vi "MaxZ_FITSstacks.vi"() -> ()   [LabVIEW 2011]
panel:
  out "error out":errorcluster
  in  "intensity scale factor":dbl=8.0
  out "plane#":i32=24
  out "Intensity Graph":u16[][](graph)
  in  "output folder for 16bit TIFs":path=path "D:/freigabe/Max"
  out "fits#":i32=365
  in  "All Files in Dir":path[](array[path])=[path "E:/Auswertung_ISS/002_2018-06-21_16-44-14/raw_I000_X0_C0.fits.EPI.fits", path "E:/Auswertung_ISS/002_2018-06-21_16-44-14/raw_I000_X0_C1.fits.EPI.fits", path "E:/Auswertung_ISS/002_2018-06-21_16-44-14/raw_I000_X0_C3.fits.EPI.fits", path "E:/Auswertung_ISS/002_2018-06-21_16-44-14/raw_I000_X1_C0.fits.EPI.fits", path "E:/Auswertung_ISS/002_2018-06-21_16-44-14/raw_I000_X1_C3.fits.EPI.fits", path "E:/Auswertung_ISS/003_2018-07-03_15-08-29/raw_I000_X0_C0.fits.EPI.fits", path "E:/Auswertung_ISS/003_2018-07-03_15-08-29/raw_I000_X0_C1.fits.EPI.fits", path "E:/Auswertung_ISS/003_2018-07-03_15-08-29/raw_I000_X0_C3.fits.EPI.fits", path "E:/Auswertung_ISS/003_2018-07-03_15-08-29/raw_I000_X1_C0.fits.EPI.fits", path "E:/Auswertung_ISS/003_2018-07-03_15-08-29/raw_I000_X1_C3.fits.EPI.fits", path "E:/Auswertung_ISS/003_2018-07-03_15-08-29/raw_I001_X1_C0.fits.EPI.fits", path "E:/Auswertung_ISS/003_2018-07-03_15-08-29/raw_I001_X1_C3.fits.EPI.fits", path "E:/Auswertung_ISS/003_2018-07-03_15-08-29/raw_I002_X1_C0.fits.EPI.fits", path "E:/Auswertung_ISS/003_2018-07-03_15-08-29/raw_I002_X1_C3.fits.EPI.fits", path "E:/Auswertung_ISS/003_2018-07-03_15-08-29/raw_I003_X1_C0.fits.EPI.fits", path "E:/Auswertung_ISS/003_2018-07-03_15-08-29/raw_I003_X1_C3.fits.EPI.fits", path "E:/Auswertung_ISS/003_2018-07-03_15-08-29/raw_I004_X1_C0.fits.EPI.fits", path "E:/Auswertung_ISS/003_2018-07-03_15-08-29/raw_I004_X1_C3.fits.EPI.fits", path "E:/Auswertung_ISS/003_2018-07-03_15-08-29/raw_I005_X1_C0.fits.EPI.fits", path "E:/Auswertung_ISS/003_2018-07-03_15-08-29/raw_I005_X1_C3.fits.EPI.fits", path "E:/Auswertung_ISS/003_2018-07-03_15-08-29/raw_I006_X1_C0.fits.EPI.fits", path "E:/Auswertung_ISS/003_2018-07-03_15-08-29/raw_I006_X1_C3.fits.EPI.fits", path "E:/Auswertung_ISS/003_2018-07-03_15-08-29/raw_I007_X1_C0.fits.EPI.fits", path "E:/Auswertung_ISS/003_2018-07-03_15-08-29/raw_I007_X1_C3.fits.EPI.fits", path "E:/Auswertung_ISS/003_2018-07-03_15-08-29/raw_I008_X1_C0.fits.EPI.fits", path "E:/Auswertung_ISS/003_2018-07-03_15-08-29/raw_I008_X1_C3.fits.EPI.fits", path "E:/Auswertung_ISS/003_2018-07-03_15-08-29/raw_I009_X0_C0.fits.EPI.fits", path "E:/Auswertung_ISS/003_2018-07-03_15-08-29/raw_I009_X0_C1.fits.EPI.fits", path "E:/Auswertung_ISS/003_2018-07-03_15-08-29/raw_I009_X0_C3.fits.EPI.fits", path "E:/Auswertung_ISS/003_2018-07-03_15-08-29/raw_I009_X1_C0.fits.EPI.fits", path "E:/Auswertung_ISS/003_2018-07-03_15-08-29/raw_I009_X1_C3.fits.EPI.fits", path "E:/Auswertung_ISS/004_2018-07-03_17-33-15/raw_I000_X0_C0.fits.EPI.fits", path "E:/Auswertung_ISS/004_2018-07-03_17-33-15/raw_I000_X0_C1.fits.EPI.fits", path "E:/Auswertung_ISS/004_2018-07-03_17-33-15/raw_I000_X0_C3.fits.EPI.fits", path "E:/Auswertung_ISS/004_2018-07-03_17-33-15/raw_I000_X1_C0.fits.EPI.fits", path "E:/Auswertung_ISS/004_2018-07-03_17-33-15/raw_I000_X1_C3.fits.EPI.fits", path "E:/Auswertung_ISS/004_2018-07-03_17-33-15/raw_I001_X1_C0.fits.EPI.fits", path "E:/Auswertung_ISS/004_2018-07-03_17-33-15/raw_I001_X1_C3.fits.EPI.fits", path "E:/Auswertung_ISS/004_2018-07-03_17-33-15/raw_I002_X1_C0.fits.EPI.fits", path "E:/Auswertung_ISS/004_2018-07-03_17-33-15/raw_I002_X1_C3.fits.EPI.fits", path "E:/Auswertung_ISS/004_2018-07-03_17-33-15/raw_I003_X1_C0.fits.EPI.fits", path "E:/Auswertung_ISS/004_2018-07-03_17-33-15/raw_I003_X1_C3.fits.EPI.fits", path "E:/Auswertung_ISS/004_2018-07-03_17-33-15/raw_I004_X1_C0.fits.EPI.fits", path "E:/Auswertung_ISS/004_2018-07-03_17-33-15/raw_I004_X1_C3.fits.EPI.fits", path "E:/Auswertung_ISS/004_2018-07-03_17-33-15/raw_I005_X1_C0.fits.EPI.fits", path "E:/Auswertung_ISS/004_2018-07-03_17-33-15/raw_I005_X1_C3.fits.EPI.fits", path "E:/Auswertung_ISS/004_2018-07-03_17-33-15/raw_I006_X1_C0.fits.EPI.fits", path "E:/Auswertung_ISS/004_2018-07-03_17-33-15/raw_I006_X1_C3.fits.EPI.fits", path "E:/Auswertung_ISS/004_2018-07-03_17-33-15/raw_I007_X1_C0.fits.EPI.fits", path "E:/Auswertung_ISS/004_2018-07-03_17-33-15/raw_I007_X1_C3.fits.EPI.fits", path "E:/Auswertung_ISS/004_2018-07-03_17-33-15/raw_I008_X1_C0.fits.EPI.fits", path "E:/Auswertung_ISS/004_2018-07-03_17-33-15/raw_I008_X1_C3.fits.EPI.fits", path "E:/Auswertung_ISS/004_2018-07-03_17-33-15/raw_I009_X1_C0.fits.EPI.fits", path "E:/Auswertung_ISS/004_2018-07-03_17-33-15/raw_I009_X1_C3.fits.EPI.fits", path "E:/Auswertung_ISS/004_2018-07-03_17-33-15/raw_I010_X1_C0.fits.EPI.fits", path "E:/Auswertung_ISS/004_2018-07-03_17-33-15/raw_I010_X1_C3.fits.EPI.fits", path "E:/Auswertung_ISS/004_2018-07-03_17-33-15/raw_I011_X1_C0.fits.EPI.fits", path "E:/Auswertung_ISS/004_2018-07-03_17-33-15/raw_I011_X1_C3.fits.EPI.fits", path "E:/Auswertung_ISS/004_2018-07-03_17-33-15/raw_I012_X1_C0.fits.EPI.fits", path "E:/Auswertung_ISS/004_2018-07-03_17-33-15/raw_I012_X1_C3.fits.EPI.fits", path "E:/Auswertung_ISS/004_2018-07-03_17-33-15/raw_I013_X1_C0.fits.EPI.fits", path "E:/Auswertung_ISS/004_2018-07-03_17-33-15/raw_I013_X1_C3.fits.EPI.fits", path "E:/Auswertung_ISS/004_2018-07-03_17-33-15/raw_I014_X1_C0.fits.EPI.fits", path "E:/Auswertung_ISS/004_2018-07-03_17-33-15/raw_I014_X1_C3.fits.EPI.fits", path "E:/Auswertung_ISS/004_2018-07-03_17-33-15/raw_I015_X1_C0.fits.EPI.fits", path "E:/Auswertung_ISS/004_2018-07-03_17-33-15/raw_I015_X1_C3.fits.EPI.fits", path "E:/Auswertung_ISS/004_2018-07-03_17-33-15/raw_I016_X1_C0.fits.EPI.fits", path "E:/Auswertung_ISS/004_2018-07-03_17-33-15/raw_I016_X1_C3.fits.EPI.fits", path "E:/Auswertung_ISS/004_2018-07-03_17-33-15/raw_I017_X1_C0.fits.EPI.fits", path "E:/Auswertung_ISS/004_2018-07-03_17-33-15/raw_I017_X1_C3.fits.EPI.fits", path "E:/Auswertung_ISS/005_2018-07-04_08-02-54/raw_I000_X0_C0.fits.EPI.fits", path "E:/Auswertung_ISS/005_2018-07-04_08-02-54/raw_I000_X0_C1.fits.EPI.fits", path "E:/Auswertung_ISS/005_2018-07-04_08-02-54/raw_I000_X0_C3.fits.EPI.fits", path "E:/Auswertung_ISS/005_2018-07-04_08-02-54/raw_I000_X1_C0.fits.EPI.fits", path "E:/Auswertung_ISS/005_2018-07-04_08-02-54/raw_I000_X1_C3.fits.EPI.fits", path "E:/Auswertung_ISS/005_2018-07-04_08-02-54/raw_I001_X1_C0.fits.EPI.fits", path "E:/Auswertung_ISS/005_2018-07-04_08-02-54/raw_I001_X1_C3.fits.EPI.fits", path "E:/Auswertung_ISS/005_2018-07-04_08-02-54/raw_I002_X1_C0.fits.EPI.fits", path "E:/Auswertung_ISS/005_2018-07-04_08-02-54/raw_I002_X1_C3.fits.EPI.fits", path "E:/Auswertung_ISS/005_2018-07-04_08-02-54/raw_I003_X1_C0.fits.EPI.fits", path "E:/Auswertung_ISS/005_2018-07-04_08-02-54/raw_I003_X1_C3.fits.EPI.fits", path "E:/Auswertung_ISS/005_2018-07-04_08-02-54/raw_I004_X1_C0.fits.EPI.fits", path "E:/Auswertung_ISS/005_2018-07-04_08-02-54/raw_I004_X1_C3.fits.EPI.fits", path "E:/Auswertung_ISS/005_2018-07-04_08-02-54/raw_I005_X1_C0.fits.EPI.fits", path "E:/Auswertung_ISS/005_2018-07-04_08-02-54/raw_I005_X1_C3.fits.EPI.fits", path "E:/Auswertung_ISS/005_2018-07-04_08-02-54/raw_I006_X1_C0.fits.EPI.fits", path "E:/Auswertung_ISS/005_2018-07-04_08-02-54/raw_I006_X1_C3.fits.EPI.fits", path "E:/Auswertung_ISS/005_2018-07-04_08-02-54/raw_I007_X1_C0.fits.EPI.fits", path "E:/Auswertung_ISS/005_2018-07-04_08-02-54/raw_I007_X1_C3.fits.EPI.fits", path "E:/Auswertung_ISS/005_2018-07-04_08-02-54/raw_I008_X1_C0.fits.EPI.fits", path "E:/Auswertung_ISS/005_2018-07-04_08-02-54/raw_I008_X1_C3.fits.EPI.fits", path "E:/Auswertung_ISS/005_2018-07-04_08-02-54/raw_I009_X1_C0.fits.EPI.fits", path "E:/Auswertung_ISS/005_2018-07-04_08-02-54/raw_I009_X1_C3.fits.EPI.fits", path "E:/Auswertung_ISS/005_2018-07-04_08-02-54/raw_I010_X1_C0.fits.EPI.fits", path "E:/Auswertung_ISS/005_2018-07-04_08-02-54/raw_I010_X1_C3.fits.EPI.fits", path "E:/Auswertung_ISS/005_2018-07-04_08-02-54/raw_I011_X1_C0.fits.EPI.fits", path "E:/Auswertung_ISS/005_2018-07-04_08-02-54/raw_I011_X1_C3.fits.EPI.fits", path "E:/Auswertung_ISS/005_2018-07-04_08-02-54/raw_I012_X1_C0.fits.EPI.fits", path "E:/Auswertung_ISS/005_2018-07-04_08-02-54/raw_I012_X1_C3.fits.EPI.fits", path "E:/Auswertung_ISS/005_2018-07-04_08-02-54/raw_I013_X1_C0.fits.EPI.fits", path "E:/Auswertung_ISS/005_2018-07-04_08-02-54/raw_I013_X1_C3.fits.EPI.fits", path "E:/Auswertung_ISS/005_2018-07-04_08-02-54/raw_I014_X1_C0.fits.EPI.fits", path "E:/Auswertung_ISS/005_2018-07-04_08-02-54/raw_I014_X1_C3.fits.EPI.fits", path "E:/Auswertung_ISS/005_2018-07-04_08-02-54/raw_I015_X1_C0.fits.EPI.fits", path "E:/Auswertung_ISS/005_2018-07-04_08-02-54/raw_I015_X1_C3.fits.EPI.fits", path "E:/Auswertung_ISS/005_2018-07-04_08-02-54/raw_I016_X1_C0.fits.EPI.fits", path "E:/Auswertung_ISS/005_2018-07-04_08-02-54/raw_I016_X1_C3.fits.EPI.fits", path "E:/Auswertung_ISS/006_2018-07-04_15-43-18/raw_I000_X0_C0.fits.EPI.fits", path "E:/Auswertung_ISS/006_2018-07-04_15-43-18/raw_I000_X0_C1.fits.EPI.fits", path "E:/Auswertung_ISS/006_2018-07-04_15-43-18/raw_I000_X0_C3.fits.EPI.fits", path "E:/Auswertung_ISS/006_2018-07-04_15-43-18/raw_I000_X1_C0.fits.EPI.fits", path "E:/Auswertung_ISS/006_2018-07-04_15-43-18/raw_I000_X1_C3.fits.EPI.fits", path "E:/Auswertung_ISS/006_2018-07-04_15-43-18/raw_I001_X1_C0.fits.EPI.fits", path "E:/Auswertung_ISS/006_2018-07-04_15-43-18/raw_I001_X1_C3.fits.EPI.fits", path "E:/Auswertung_ISS/006_2018-07-04_15-43-18/raw_I002_X1_C0.fits.EPI.fits", path "E:/Auswertung_ISS/006_2018-07-04_15-43-18/raw_I002_X1_C3.fits.EPI.fits", path "E:/Auswertung_ISS/006_2018-07-04_15-43-18/raw_I003_X1_C0.fits.EPI.fits", path "E:/Auswertung_ISS/006_2018-07-04_15-43-18/raw_I003_X1_C3.fits.EPI.fits", path "E:/Auswertung_ISS/007_2018-07-04_16-44-22/raw_I000_X0_C0.fits.EPI.fits", path "E:/Auswertung_ISS/007_2018-07-04_16-44-22/raw_I000_X0_C1.fits.EPI.fits", path "E:/Auswertung_ISS/007_2018-07-04_16-44-22/raw_I000_X0_C3.fits.EPI.fits", path "E:/Auswertung_ISS/007_2018-07-04_16-44-22/raw_I000_X1_C0.fits.EPI.fits", path "E:/Auswertung_ISS/007_2018-07-04_16-44-22/raw_I000_X1_C3.fits.EPI.fits", path "E:/Auswertung_ISS/007_2018-07-04_16-44-22/raw_I001_X1_C0.fits.EPI.fits", path "E:/Auswertung_ISS/007_2018-07-04_16-44-22/raw_I001_X1_C3.fits.EPI.fits", path "E:/Auswertung_ISS/007_2018-07-04_16-44-22/raw_I002_X1_C0.fits.EPI.fits", path "E:/Auswertung_ISS/007_2018-07-04_16-44-22/raw_I002_X1_C3.fits.EPI.fits", path "E:/Auswertung_ISS/007_2018-07-04_16-44-22/raw_I003_X1_C0.fits.EPI.fits", path "E:/Auswertung_ISS/007_2018-07-04_16-44-22/raw_I003_X1_C3.fits.EPI.fits", path "E:/Auswertung_ISS/007_2018-07-04_16-44-22/raw_I004_X1_C0.fits.EPI.fits", path "E:/Auswertung_ISS/007_2018-07-04_16-44-22/raw_I004_X1_C3.fits.EPI.fits", path "E:/Auswertung_ISS/007_2018-07-04_16-44-22/raw_I005_X1_C0.fits.EPI.fits", path "E:/Auswertung_ISS/007_2018-07-04_16-44-22/raw_I005_X1_C3.fits.EPI.fits", path "E:/Auswertung_ISS/007_2018-07-04_16-44-22/raw_I006_X1_C0.fits.EPI.fits", path "E:/Auswertung_ISS/007_2018-07-04_16-44-22/raw_I006_X1_C3.fits.EPI.fits", path "E:/Auswertung_ISS/007_2018-07-04_16-44-22/raw_I007_X1_C0.fits.EPI.fits", path "E:/Auswertung_ISS/007_2018-07-04_16-44-22/raw_I007_X1_C3.fits.EPI.fits", path "E:/Auswertung_ISS/007_2018-07-04_16-44-22/raw_I008_X1_C0.fits.EPI.fits", path "E:/Auswertung_ISS/007_2018-07-04_16-44-22/raw_I008_X1_C3.fits.EPI.fits", path "E:/Auswertung_ISS/007_2018-07-04_16-44-22/raw_I009_X1_C0.fits.EPI.fits", path "E:/Auswertung_ISS/007_2018-07-04_16-44-22/raw_I009_X1_C3.fits.EPI.fits", path "E:/Auswertung_ISS/007_2018-07-04_16-44-22/raw_I010_X1_C0.fits.EPI.fits", path "E:/Auswertung_ISS/007_2018-07-04_16-44-22/raw_I010_X1_C3.fits.EPI.fits", path "E:/Auswertung_ISS/007_2018-07-04_16-44-22/raw_I011_X1_C0.fits.EPI.fits", path "E:/Auswertung_ISS/007_2018-07-04_16-44-22/raw_I011_X1_C3.fits.EPI.fits", path "E:/Auswertung_ISS/007_2018-07-04_16-44-22/raw_I012_X1_C0.fits.EPI.fits", path "E:/Auswertung_ISS/007_2018-07-04_16-44-22/raw_I012_X1_C3.fits.EPI.fits", path "E:/Auswertung_ISS/007_2018-07-04_16-44-22/raw_I013_X1_C0.fits.EPI.fits", path "E:/Auswertung_ISS/007_2018-07-04_16-44-22/raw_I013_X1_C3.fits.EPI.fits", path "E:/Auswertung_ISS/007_2018-07-04_16-44-22/raw_I014_X1_C0.fits.EPI.fits", path "E:/Auswertung_ISS/007_2018-07-04_16-44-22/raw_I014_X1_C3.fits.EPI.fits", path "E:/Auswertung_ISS/007_2018-07-04_16-44-22/raw_I015_X1_C0.fits.EPI.fits", path "E:/Auswertung_ISS/007_2018-07-04_16-44-22/raw_I015_X1_C3.fits.EPI.fits", path "E:/Auswertung_ISS/007_2018-07-04_16-44-22/raw_I016_X1_C0.fits.EPI.fits", path "E:/Auswertung_ISS/007_2018-07-04_16-44-22/raw_I016_X1_C3.fits.EPI.fits", path "E:/Auswertung_ISS/007_2018-07-04_16-44-22/raw_I017_X1_C0.fits.EPI.fits", path "E:/Auswertung_ISS/007_2018-07-04_16-44-22/raw_I017_X1_C3.fits.EPI.fits", path "E:/Auswertung_ISS/008_2018-07-05_08-02-52/raw_I000_X0_C0.fits.EPI.fits", path "E:/Auswertung_ISS/008_2018-07-05_08-02-52/raw_I000_X0_C1.fits.EPI.fits", path "E:/Auswertung_ISS/008_2018-07-05_08-02-52/raw_I000_X0_C3.fits.EPI.fits", path "E:/Auswertung_ISS/008_2018-07-05_08-02-52/raw_I000_X1_C0.fits.EPI.fits", path "E:/Auswertung_ISS/008_2018-07-05_08-02-52/raw_I000_X1_C3.fits.EPI.fits", path "E:/Auswertung_ISS/008_2018-07-05_08-02-52/raw_I001_X1_C0.fits.EPI.fits", path "E:/Auswertung_ISS/008_2018-07-05_08-02-52/raw_I001_X1_C3.fits.EPI.fits", path "E:/Auswertung_ISS/008_2018-07-05_08-02-52/raw_I002_X1_C0.fits.EPI.fits", path "E:/Auswertung_ISS/008_2018-07-05_08-02-52/raw_I002_X1_C3.fits.EPI.fits", path "E:/Auswertung_ISS/008_2018-07-05_08-02-52/raw_I003_X1_C0.fits.EPI.fits", path "E:/Auswertung_ISS/008_2018-07-05_08-02-52/raw_I003_X1_C3.fits.EPI.fits", path "E:/Auswertung_ISS/008_2018-07-05_08-02-52/raw_I004_X1_C0.fits.EPI.fits", path "E:/Auswertung_ISS/008_2018-07-05_08-02-52/raw_I004_X1_C3.fits.EPI.fits", path "E:/Auswertung_ISS/008_2018-07-05_08-02-52/raw_I005_X1_C0.fits.EPI.fits", path "E:/Auswertung_ISS/008_2018-07-05_08-02-52/raw_I005_X1_C3.fits.EPI.fits", path "E:/Auswertung_ISS/008_2018-07-05_08-02-52/raw_I006_X1_C0.fits.EPI.fits", path "E:/Auswertung_ISS/008_2018-07-05_08-02-52/raw_I006_X1_C3.fits.EPI.fits", path "E:/Auswertung_ISS/008_2018-07-05_08-02-52/raw_I007_X1_C0.fits.EPI.fits", path "E:/Auswertung_ISS/008_2018-07-05_08-02-52/raw_I007_X1_C3.fits.EPI.fits", path "E:/Auswertung_ISS/008_2018-07-05_08-02-52/raw_I008_X1_C0.fits.EPI.fits", path "E:/Auswertung_ISS/008_2018-07-05_08-02-52/raw_I008_X1_C3.fits.EPI.fits", path "E:/Auswertung_ISS/008_2018-07-05_08-02-52/raw_I009_X1_C0.fits.EPI.fits", path "E:/Auswertung_ISS/008_2018-07-05_08-02-52/raw_I009_X1_C3.fits.EPI.fits", path "E:/Auswertung_ISS/008_2018-07-05_08-02-52/raw_I010_X1_C0.fits.EPI.fits", path "E:/Auswertung_ISS/008_2018-07-05_08-02-52/raw_I010_X1_C3.fits.EPI.fits", path "E:/Auswertung_ISS/008_2018-07-05_08-02-52/raw_I011_X1_C0.fits.EPI.fits", path "E:/Auswertung_ISS/008_2018-07-05_08-02-52/raw_I011_X1_C3.fits.EPI.fits", path "E:/Auswertung_ISS/008_2018-07-05_08-02-52/raw_I012_X1_C0.fits.EPI.fits", path "E:/Auswertung_ISS/008_2018-07-05_08-02-52/raw_I012_X1_C3.fits.EPI.fits", path "E:/Auswertung_ISS/008_2018-07-05_08-02-52/raw_I013_X1_C0.fits.EPI.fits", path "E:/Auswertung_ISS/008_2018-07-05_08-02-52/raw_I013_X1_C3.fits.EPI.fits", path "E:/Auswertung_ISS/008_2018-07-05_08-02-52/raw_I014_X1_C0.fits.EPI.fits", path "E:/Auswertung_ISS/008_2018-07-05_08-02-52/raw_I014_X1_C3.fits.EPI.fits", path "E:/Auswertung_ISS/008_2018-07-05_08-02-52/raw_I015_X1_C0.fits.EPI.fits", path "E:/Auswertung_ISS/008_2018-07-05_08-02-52/raw_I015_X1_C3.fits.EPI.fits", path "E:/Auswertung_ISS/008_2018-07-05_08-02-52/raw_I016_X1_C0.fits.EPI.fits", path "E:/Auswertung_ISS/008_2018-07-05_08-02-52/raw_I016_X1_C3.fits.EPI.fits", path "E:/Auswertung_ISS/008_2018-07-05_08-02-52/raw_I017_X1_C0.fits.EPI.fits", path "E:/Auswertung_ISS/008_2018-07-05_08-02-52/raw_I017_X1_C3.fits.EPI.fits", path "E:/Auswertung_ISS/009_2018-07-05_20-57-36/raw_I000_X0_C0.fits.EPI.fits", path "E:/Auswertung_ISS/009_2018-07-05_20-57-36/raw_I000_X0_C1.fits.EPI.fits", path "E:/Auswertung_ISS/009_2018-07-05_20-57-36/raw_I000_X0_C3.fits.EPI.fits", path "E:/Auswertung_ISS/009_2018-07-05_20-57-36/raw_I000_X1_C3.fits.EPI.fits", path "E:/Auswertung_ISS/009_2018-07-05_20-57-36/raw_I001_X1_C3.fits.EPI.fits", path "E:/Auswertung_ISS/009_2018-07-05_20-57-36/raw_I002_X1_C3.fits.EPI.fits", path "E:/Auswertung_ISS/009_2018-07-05_20-57-36/raw_I003_X1_C3.fits.EPI.fits", path "E:/Auswertung_ISS/009_2018-07-05_20-57-36/raw_I004_X1_C3.fits.EPI.fits", path "E:/Auswertung_ISS/009_2018-07-05_20-57-36/raw_I005_X1_C3.fits.EPI.fits", path "E:/Auswertung_ISS/009_2018-07-05_20-57-36/raw_I006_X1_C3.fits.EPI.fits", path "E:/Auswertung_ISS/009_2018-07-05_20-57-36/raw_I007_X1_C3.fits.EPI.fits", path "E:/Auswertung_ISS/009_2018-07-05_20-57-36/raw_I008_X1_C3.fits.EPI.fits", path "E:/Auswertung_ISS/009_2018-07-05_20-57-36/raw_I009_X1_C3.fits.EPI.fits", path "E:/Auswertung_ISS/009_2018-07-05_20-57-36/raw_I010_X1_C3.fits.EPI.fits", path "E:/Auswertung_ISS/009_2018-07-05_20-57-36/raw_I011_X1_C3.fits.EPI.fits", path "E:/Auswertung_ISS/010_2018-07-06_17-20-26/raw_I000_X0_C0.fits.EPI.fits", path "E:/Auswertung_ISS/010_2018-07-06_17-20-26/raw_I000_X0_C1.fits.EPI.fits", path "E:/Auswertung_ISS/010_2018-07-06_17-20-26/raw_I000_X0_C3.fits.EPI.fits", path "E:/Auswertung_ISS/010_2018-07-06_17-20-26/raw_I000_X1_C3.fits.EPI.fits", path "E:/Auswertung_ISS/010_2018-07-06_17-20-26/raw_I001_X0_C0.fits.EPI.fits", path "E:/Auswertung_ISS/010_2018-07-06_17-20-26/raw_I001_X0_C1.fits.EPI.fits", path "E:/Auswertung_ISS/010_2018-07-06_17-20-26/raw_I001_X0_C3.fits.EPI.fits", path "E:/Auswertung_ISS/011_2018-07-06_17-40-54/raw_I000_X0_C0.fits.EPI.fits", path "E:/Auswertung_ISS/011_2018-07-06_17-40-54/raw_I000_X0_C1.fits.EPI.fits", path "E:/Auswertung_ISS/011_2018-07-06_17-40-54/raw_I000_X0_C3.fits.EPI.fits", path "E:/Auswertung_ISS/011_2018-07-06_17-40-54/raw_I000_X1_C3.fits.EPI.fits", path "E:/Auswertung_ISS/011_2018-07-06_17-40-54/raw_I001_X1_C3.fits.EPI.fits", path "E:/Auswertung_ISS/011_2018-07-06_17-40-54/raw_I002_X1_C3.fits.EPI.fits", path "E:/Auswertung_ISS/011_2018-07-06_17-40-54/raw_I003_X1_C3.fits.EPI.fits", path "E:/Auswertung_ISS/011_2018-07-06_17-40-54/raw_I004_X1_C3.fits.EPI.fits", path "E:/Auswertung_ISS/011_2018-07-06_17-40-54/raw_I005_X1_C3.fits.EPI.fits", path "E:/Auswertung_ISS/011_2018-07-06_17-40-54/raw_I006_X1_C3.fits.EPI.fits", path "E:/Auswertung_ISS/011_2018-07-06_17-40-54/raw_I007_X1_C3.fits.EPI.fits", path "E:/Auswertung_ISS/011_2018-07-06_17-40-54/raw_I008_X1_C3.fits.EPI.fits", path "E:/Auswertung_ISS/012_2018-07-07_01-02-54/raw_I000_X0_C0.fits.EPI.fits", path "E:/Auswertung_ISS/012_2018-07-07_01-02-54/raw_I000_X0_C1.fits.EPI.fits", path "E:/Auswertung_ISS/012_2018-07-07_01-02-54/raw_I000_X0_C3.fits.EPI.fits", path "E:/Auswertung_ISS/012_2018-07-07_01-02-54/raw_I000_X1_C3.fits.EPI.fits", path "E:/Auswertung_ISS/012_2018-07-07_01-02-54/raw_I001_X1_C3.fits.EPI.fits", path "E:/Auswertung_ISS/012_2018-07-07_01-02-54/raw_I002_X1_C3.fits.EPI.fits", path "E:/Auswertung_ISS/012_2018-07-07_01-02-54/raw_I003_X1_C3.fits.EPI.fits", path "E:/Auswertung_ISS/012_2018-07-07_01-02-54/raw_I004_X1_C3.fits.EPI.fits", path "E:/Auswertung_ISS/012_2018-07-07_01-02-54/raw_I005_X1_C3.fits.EPI.fits", path "E:/Auswertung_ISS/012_2018-07-07_01-02-54/raw_I006_X1_C3.fits.EPI.fits", path "E:/Auswertung_ISS/013_2018-07-07_08-02-53/raw_I000_X0_C0.fits.EPI.fits", path "E:/Auswertung_ISS/013_2018-07-07_08-02-53/raw_I000_X0_C1.fits.EPI.fits", path "E:/Auswertung_ISS/013_2018-07-07_08-02-53/raw_I000_X0_C3.fits.EPI.fits", path "E:/Auswertung_ISS/013_2018-07-07_08-02-53/raw_I000_X1_C0.fits.EPI.fits", path "E:/Auswertung_ISS/013_2018-07-07_08-02-53/raw_I000_X1_C3.fits.EPI.fits", path "E:/Auswertung_ISS/013_2018-07-07_08-02-53/raw_I001_X1_C0.fits.EPI.fits", path "E:/Auswertung_ISS/013_2018-07-07_08-02-53/raw_I001_X1_C3.fits.EPI.fits", path "E:/Auswertung_ISS/013_2018-07-07_08-02-53/raw_I002_X1_C0.fits.EPI.fits", path "E:/Auswertung_ISS/013_2018-07-07_08-02-53/raw_I002_X1_C3.fits.EPI.fits", path "E:/Auswertung_ISS/013_2018-07-07_08-02-53/raw_I003_X1_C0.fits.EPI.fits", path "E:/Auswertung_ISS/013_2018-07-07_08-02-53/raw_I003_X1_C3.fits.EPI.fits", path "E:/Auswertung_ISS/013_2018-07-07_08-02-53/raw_I004_X1_C0.fits.EPI.fits", path "E:/Auswertung_ISS/013_2018-07-07_08-02-53/raw_I004_X1_C3.fits.EPI.fits", path "E:/Auswertung_ISS/013_2018-07-07_08-02-53/raw_I005_X1_C0.fits.EPI.fits", path "E:/Auswertung_ISS/013_2018-07-07_08-02-53/raw_I005_X1_C3.fits.EPI.fits", path "E:/Auswertung_ISS/013_2018-07-07_08-02-53/raw_I006_X1_C0.fits.EPI.fits", path "E:/Auswertung_ISS/013_2018-07-07_08-02-53/raw_I006_X1_C3.fits.EPI.fits", path "E:/Auswertung_ISS/013_2018-07-07_08-02-53/raw_I007_X1_C0.fits.EPI.fits", path "E:/Auswertung_ISS/013_2018-07-07_08-02-53/raw_I007_X1_C3.fits.EPI.fits", path "E:/Auswertung_ISS/013_2018-07-07_08-02-53/raw_I008_X1_C0.fits.EPI.fits", path "E:/Auswertung_ISS/013_2018-07-07_08-02-53/raw_I008_X1_C3.fits.EPI.fits", path "E:/Auswertung_ISS/013_2018-07-07_08-02-53/raw_I009_X1_C0.fits.EPI.fits", path "E:/Auswertung_ISS/013_2018-07-07_08-02-53/raw_I009_X1_C3.fits.EPI.fits", path "E:/Auswertung_ISS/013_2018-07-07_08-02-53/raw_I010_X1_C0.fits.EPI.fits", path "E:/Auswertung_ISS/013_2018-07-07_08-02-53/raw_I010_X1_C3.fits.EPI.fits", path "E:/Auswertung_ISS/013_2018-07-07_08-02-53/raw_I011_X1_C0.fits.EPI.fits", path "E:/Auswertung_ISS/013_2018-07-07_08-02-53/raw_I011_X1_C3.fits.EPI.fits", path "E:/Auswertung_ISS/013_2018-07-07_08-02-53/raw_I012_X1_C0.fits.EPI.fits", path "E:/Auswertung_ISS/013_2018-07-07_08-02-53/raw_I012_X1_C3.fits.EPI.fits", path "E:/Auswertung_ISS/013_2018-07-07_08-02-53/raw_I013_X1_C0.fits.EPI.fits", path "E:/Auswertung_ISS/013_2018-07-07_08-02-53/raw_I013_X1_C3.fits.EPI.fits", path "E:/Auswertung_ISS/013_2018-07-07_08-02-53/raw_I014_X1_C0.fits.EPI.fits", path "E:/Auswertung_ISS/013_2018-07-07_08-02-53/raw_I014_X1_C3.fits.EPI.fits", path "E:/Auswertung_ISS/013_2018-07-07_08-02-53/raw_I015_X1_C0.fits.EPI.fits", path "E:/Auswertung_ISS/013_2018-07-07_08-02-53/raw_I015_X1_C3.fits.EPI.fits", path "E:/Auswertung_ISS/013_2018-07-07_08-02-53/raw_I016_X1_C0.fits.EPI.fits", path "E:/Auswertung_ISS/013_2018-07-07_08-02-53/raw_I016_X1_C3.fits.EPI.fits", path "E:/Auswertung_ISS/013_2018-07-07_08-02-53/raw_I017_X1_C0.fits.EPI.fits", path "E:/Auswertung_ISS/013_2018-07-07_08-02-53/raw_I017_X1_C3.fits.EPI.fits", path "E:/Auswertung_ISS/013_2018-07-07_08-02-53/raw_I018_X1_C0.fits.EPI.fits", path "E:/Auswertung_ISS/013_2018-07-07_08-02-53/raw_I018_X1_C3.fits.EPI.fits", path "E:/Auswertung_ISS/013_2018-07-07_08-02-53/raw_I019_X1_C0.fits.EPI.fits", path "E:/Auswertung_ISS/013_2018-07-07_08-02-53/raw_I019_X1_C3.fits.EPI.fits", path "E:/Auswertung_ISS/013_2018-07-07_08-02-53/raw_I020_X1_C0.fits.EPI.fits", path "E:/Auswertung_ISS/013_2018-07-07_08-02-53/raw_I020_X1_C3.fits.EPI.fits", path "E:/Auswertung_ISS/013_2018-07-07_08-02-53/raw_I021_X1_C0.fits.EPI.fits", path "E:/Auswertung_ISS/013_2018-07-07_08-02-53/raw_I021_X1_C3.fits.EPI.fits", path "E:/Auswertung_ISS/013_2018-07-07_08-02-53/raw_I022_X1_C0.fits.EPI.fits", path "E:/Auswertung_ISS/013_2018-07-07_08-02-53/raw_I022_X1_C3.fits.EPI.fits", path "E:/Auswertung_ISS/013_2018-07-07_08-02-53/raw_I023_X1_C0.fits.EPI.fits", path "E:/Auswertung_ISS/013_2018-07-07_08-02-53/raw_I023_X1_C3.fits.EPI.fits", path "E:/Auswertung_ISS/013_2018-07-07_08-02-53/raw_I024_X1_C0.fits.EPI.fits", path "E:/Auswertung_ISS/013_2018-07-07_08-02-53/raw_I024_X1_C3.fits.EPI.fits", path "E:/Auswertung_ISS/013_2018-07-07_08-02-53/raw_I025_X1_C0.fits.EPI.fits", path "E:/Auswertung_ISS/013_2018-07-07_08-02-53/raw_I025_X1_C3.fits.EPI.fits", path "E:/Auswertung_ISS/013_2018-07-07_08-02-53/raw_I026_X1_C0.fits.EPI.fits", path "E:/Auswertung_ISS/013_2018-07-07_08-02-53/raw_I026_X1_C3.fits.EPI.fits", path "E:/Auswertung_ISS/013_2018-07-07_08-02-53/raw_I027_X1_C0.fits.EPI.fits", path "E:/Auswertung_ISS/013_2018-07-07_08-02-53/raw_I027_X1_C3.fits.EPI.fits", path "E:/Auswertung_ISS/013_2018-07-07_08-02-53/raw_I028_X1_C0.fits.EPI.fits", path "E:/Auswertung_ISS/013_2018-07-07_08-02-53/raw_I028_X1_C3.fits.EPI.fits", path "E:/Auswertung_ISS/013_2018-07-07_08-02-53/raw_I029_X1_C0.fits.EPI.fits", path "E:/Auswertung_ISS/013_2018-07-07_08-02-53/raw_I029_X1_C3.fits.EPI.fits", path "E:/Auswertung_ISS/014_2018-07-16_17-53-52/raw_I000_X0_C0.fits.EPI.fits", path "E:/Auswertung_ISS/014_2018-07-16_17-53-52/raw_I000_X0_C1.fits.EPI.fits", path "E:/Auswertung_ISS/014_2018-07-16_17-53-52/raw_I000_X0_C3.fits.EPI.fits", path "E:/Auswertung_ISS/014_2018-07-16_17-53-52/raw_I000_X1_C0.fits.EPI.fits", path "E:/Auswertung_ISS/014_2018-07-16_17-53-52/raw_I000_X1_C3.fits.EPI.fits", path "E:/Auswertung_ISS/014_2018-07-16_17-53-52/raw_I001_X1_C0.fits.EPI.fits", path "E:/Auswertung_ISS/014_2018-07-16_17-53-52/raw_I001_X1_C3.fits.EPI.fits", path "E:/Auswertung_ISS/014_2018-07-16_17-53-52/raw_I002_X1_C0.fits.EPI.fits", path "E:/Auswertung_ISS/014_2018-07-16_17-53-52/raw_I002_X1_C3.fits.EPI.fits", path "E:/Auswertung_ISS/014_2018-07-16_17-53-52/raw_I003_X1_C0.fits.EPI.fits", path "E:/Auswertung_ISS/014_2018-07-16_17-53-52/raw_I003_X1_C3.fits.EPI.fits", path "E:/Auswertung_ISS/014_2018-07-16_17-53-52/raw_I004_X1_C0.fits.EPI.fits", path "E:/Auswertung_ISS/014_2018-07-16_17-53-52/raw_I004_X1_C3.fits.EPI.fits", path "E:/Auswertung_ISS/014_2018-07-16_17-53-52/raw_I005_X1_C0.fits.EPI.fits", path "E:/Auswertung_ISS/014_2018-07-16_17-53-52/raw_I005_X1_C3.fits.EPI.fits", path "E:/Auswertung_ISS/014_2018-07-16_17-53-52/raw_I006_X1_C0.fits.EPI.fits", path "E:/Auswertung_ISS/014_2018-07-16_17-53-52/raw_I006_X1_C3.fits.EPI.fits", path "E:/Auswertung_ISS/014_2018-07-16_17-53-52/raw_I007_X1_C0.fits.EPI.fits", path "E:/Auswertung_ISS/014_2018-07-16_17-53-52/raw_I007_X1_C3.fits.EPI.fits", path "E:/Auswertung_ISS/014_2018-07-16_17-53-52/raw_I008_X1_C0.fits.EPI.fits", path "E:/Auswertung_ISS/014_2018-07-16_17-53-52/raw_I008_X1_C3.fits.EPI.fits", path "E:/Auswertung_ISS/014_2018-07-16_17-53-52/raw_I009_X1_C0.fits.EPI.fits", path "E:/Auswertung_ISS/014_2018-07-16_17-53-52/raw_I009_X1_C3.fits.EPI.fits", path "E:/Auswertung_ISS/014_2018-07-16_17-53-52/raw_I010_X1_C0.fits.EPI.fits", path "E:/Auswertung_ISS/014_2018-07-16_17-53-52/raw_I010_X1_C3.fits.EPI.fits", path "E:/Auswertung_ISS/014_2018-07-16_17-53-52/raw_I011_X1_C0.fits.EPI.fits", path "E:/Auswertung_ISS/014_2018-07-16_17-53-52/raw_I011_X1_C3.fits.EPI.fits", path "E:/Auswertung_ISS/014_2018-07-16_17-53-52/raw_I012_X1_C0.fits.EPI.fits", path "E:/Auswertung_ISS/014_2018-07-16_17-53-52/raw_I012_X1_C3.fits.EPI.fits", path "E:/Auswertung_ISS/014_2018-07-16_17-53-52/raw_I013_X1_C0.fits.EPI.fits", path "E:/Auswertung_ISS/014_2018-07-16_17-53-52/raw_I013_X1_C3.fits.EPI.fits", path "E:/Auswertung_ISS/014_2018-07-16_17-53-52/raw_I014_X1_C0.fits.EPI.fits", path "E:/Auswertung_ISS/014_2018-07-16_17-53-52/raw_I014_X1_C3.fits.EPI.fits", path "E:/Auswertung_ISS/014_2018-07-16_17-53-52/raw_I015_X1_C0.fits.EPI.fits", path "E:/Auswertung_ISS/014_2018-07-16_17-53-52/raw_I015_X1_C3.fits.EPI.fits", path "E:/Auswertung_ISS/014_2018-07-16_17-53-52/raw_I016_X1_C0.fits.EPI.fits", path "E:/Auswertung_ISS/014_2018-07-16_17-53-52/raw_I016_X1_C3.fits.EPI.fits", path "E:/Auswertung_ISS/014_2018-07-16_17-53-52/raw_I017_X1_C0.fits.EPI.fits", path "E:/Auswertung_ISS/014_2018-07-16_17-53-52/raw_I017_X1_C3.fits.EPI.fits", path "E:/Auswertung_ISS/014_2018-07-16_17-53-52/raw_I018_X1_C0.fits.EPI.fits", path "E:/Auswertung_ISS/014_2018-07-16_17-53-52/raw_I018_X1_C3.fits.EPI.fits", path "E:/Auswertung_ISS/014_2018-07-16_17-53-52/raw_I019_X1_C0.fits.EPI.fits", path "E:/Auswertung_ISS/014_2018-07-16_17-53-52/raw_I019_X1_C3.fits.EPI.fits", path "E:/Auswertung_ISS/014_2018-07-16_17-53-52/raw_I020_X1_C0.fits.EPI.fits", path "E:/Auswertung_ISS/014_2018-07-16_17-53-52/raw_I020_X1_C3.fits.EPI.fits", path "E:/Auswertung_ISS/014_2018-07-16_17-53-52/raw_I021_X1_C0.fits.EPI.fits", path "E:/Auswertung_ISS/014_2018-07-16_17-53-52/raw_I021_X1_C3.fits.EPI.fits", path "E:/Auswertung_ISS/014_2018-07-16_17-53-52/raw_I022_X1_C0.fits.EPI.fits", path "E:/Auswertung_ISS/014_2018-07-16_17-53-52/raw_I022_X1_C3.fits.EPI.fits", path "E:/Auswertung_ISS/014_2018-07-16_17-53-52/raw_I023_X1_C0.fits.EPI.fits", path "E:/Auswertung_ISS/014_2018-07-16_17-53-52/raw_I023_X1_C3.fits.EPI.fits", path "E:/Auswertung_ISS/014_2018-07-16_17-53-52/raw_I024_X1_C0.fits.EPI.fits", path "E:/Auswertung_ISS/014_2018-07-16_17-53-52/raw_I024_X1_C3.fits.EPI.fits", path "E:/Auswertung_ISS/014_2018-07-16_17-53-52/raw_I025_X1_C0.fits.EPI.fits", path "E:/Auswertung_ISS/014_2018-07-16_17-53-52/raw_I025_X1_C3.fits.EPI.fits", path "E:/Auswertung_ISS/014_2018-07-16_17-53-52/raw_I026_X1_C0.fits.EPI.fits", path "E:/Auswertung_ISS/014_2018-07-16_17-53-52/raw_I026_X1_C3.fits.EPI.fits", path "E:/Auswertung_ISS/014_2018-07-16_17-53-52/raw_I027_X1_C0.fits.EPI.fits", path "E:/Auswertung_ISS/014_2018-07-16_17-53-52/raw_I027_X1_C3.fits.EPI.fits", path "E:/Auswertung_ISS/014_2018-07-16_17-53-52/raw_I028_X1_C0.fits.EPI.fits", path "E:/Auswertung_ISS/014_2018-07-16_17-53-52/raw_I028_X1_C3.fits.EPI.fits", path "E:/Auswertung_ISS/014_2018-07-16_17-53-52/raw_I029_X1_C0.fits.EPI.fits", path "E:/Auswertung_ISS/014_2018-07-16_17-53-52/raw_I029_X1_C3.fits.EPI.fits"]
  # "use Recusrive File List"
  # "epi ~65000/8000= 8\nSIM ~65000/2000=32"
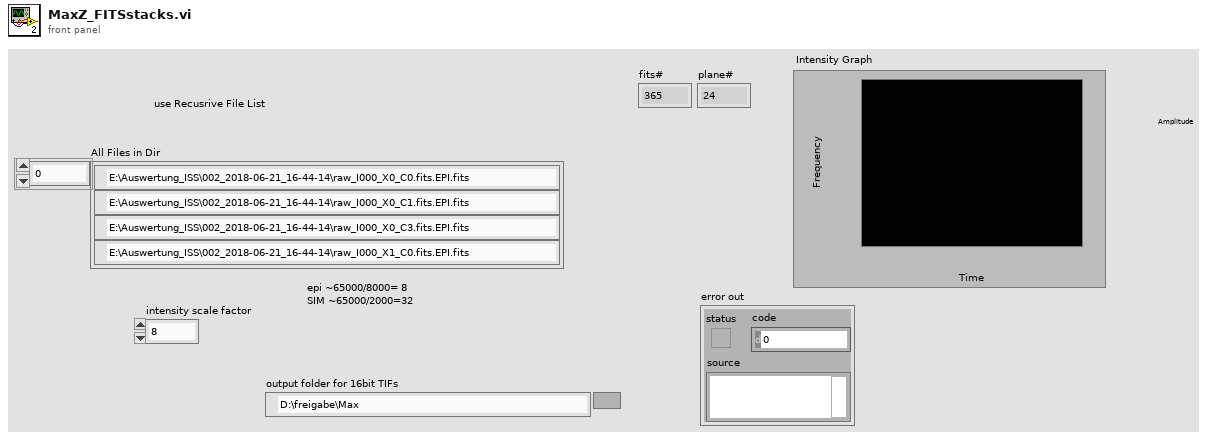
[diagram p1: front panel]
types:
  T1 = cluster{"fits refnum":refnum<file>, "Byte-Reihenfolge (0:Big-Endian, 2:LSB)":enum16{"big-endian, network order", "native, host order", "little-endian"}}
  T2 = cluster{"BITPIX":i16, "NAXIS":i16, "NAXIS1":u16, "NAXIS2":u16, "NAXIS3":u16, "BZERO":dbl, "BSCALE":dbl}
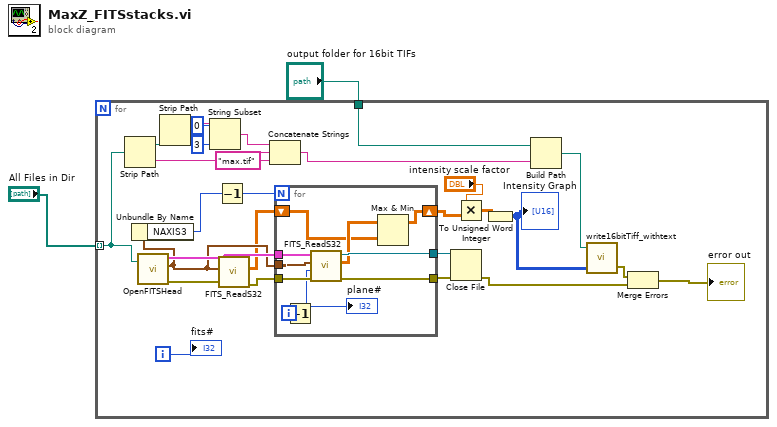
[diagram p0: block diagram]
diagram:
  n1 = for {
    tunnel: "All Files in Dir" -> [w19] mode=indexing
    tunnel: "output folder for 16bit TIFs" -> [w15]
    i -> [w30]
    n2 = Strip Path(path=w19) -> (stripped path=w7:path, name=w18:string)
    n3 = call "OpenFITSHead.vi"("file path"=w19) -> ("FITS file"=w25:T1, "FITS"=w24:T2, "error out"=w22:errorcluster)  [unwired: 2 in]
    n4 = Unbundle By Name(w24) -> ("NAXIS3"=w29:u16)
    n5 = Strip Path(path=w7) -> (name=w6:string)  [unwired: 1 out]
    n6 = String Subset(string=w6, offset (0)=0, length (rest)=3 ("length (rest)")) -> (substring=w3:string)
    n7 = Decrement(x=w29) -> (x-1=w20:u16)
    n8 = call "FITS_ReadS32.vi"("error in (no error)"=w22, "FITS"=w24, "FITS file"=w25) -> ("error out"=w21:errorcluster, "Array"=w23:sgl[][])  [unwired: 6 in, 1 out]
    n9 = Concatenate Strings(w3, w18, "max.tif" ("string")) -> (w16:string)
    n10 = for {
      N: w20 -> [_]
      tunnel: w25 -> [w40]
      tunnel: w21 -> [w39]
      tunnel: w24 -> [w38]
      tunnel: [w36] -> w28
      tunnel: [w35] -> w27
      shift-right: [w33] -> w26
      shift-left: w23 -> [w32]
      i -> [w37]
      n11 = Increment(x=w37) -> (x+1=w31:i32)
      "plane#" <- w31
      n12 = call "FITS_ReadS32.vi"("error in (no error)"=w39, "Plane# (0..n-1)"=w31, "FITS"=w38, "FITS file"=w40) -> ("error out"=w35:errorcluster, "Array"=w34:sgl[][], "Byte Stream File out"=w36:refnum<file>)  [unwired: 5 in]
      n13 = Max & Min(x=w34, y=w32) -> (max(x,y)=w33:sgl[][])  [unwired: 1 out]
    }
    n14 = Close File(refnum=w28, error in=w27) -> (error out=w9:errorcluster)  [unwired: 1 out]
    n15 = Multiply(x="intensity scale factor", y=w26) -> (x*y=w14:dbl[][])
    n16 = To Unsigned Word Integer(number=w14) -> (unsigned 16bit integer=w12:u16[][])
    "Intensity Graph" <- w12
    n17 = Build Path(base path=w15, name or relative path=w16) -> (appended path=w11:path)
    n18 = call "write16bitTiff_withtext.vi"("16-bit pixmap x, y"=w12, "file path"=w11) -> ("error out"=w10:errorcluster)  [unwired: 2 in]
    n19 = Merge Errors(w10, w9) -> (→"error out":errorcluster)
    "fits#" <- w30
  }
